vi "ComboBox.vi"(2 "Item To Select":string, 3 "Combo Box In":string(combo)="Value1") -> (0 "Combo Box Out":string(combo)="Value1", 1 "Selected Item In Input Combo Box":string)   [LabVIEW 2010]
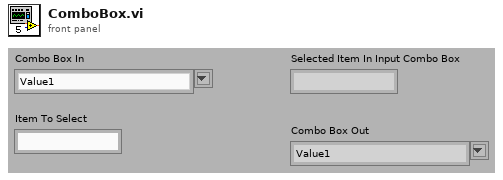
[diagram p1: front panel]
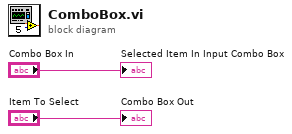
[diagram p0: block diagram]
diagram:
  "Selected Item In Input Combo Box" <- "Combo Box In"
  "Combo Box Out" <- "Item To Select"
